vi "Bridge - Continuous Input.vi"() -> ()   [LabVIEW 2021]
doc: "This example demonstrates how to continuously acquire buffered bridge measurements (force/pressure/torque) using a DAQmx device.\n\nFor instructions on how to connect your signals to the DAQ device, refer to your device documentation."
uses:
  <vilib>/Utility/error.llb/DialogType.ctl
  <vilib>/DAQmx/read.llb/DAQmx Read (Analog 1D Wfm NChan NSamp).vi
  <vilib>/DAQmx/create/channels.llb/DAQmx Create Channel (AI-Force-Bridge-Two-Point-Linear).vi
  <vilib>/DAQmx/create/channels.llb/DAQmx Create Channel (AI-Force-Bridge-Table).vi
  <vilib>/DAQmx/create/channels.llb/DAQmx Create Channel (AI-Force-Bridge-Polynomial).vi
  <vilib>/DAQmx/create/channels.llb/DAQmx Create Channel (AI-Pressure-Bridge-Two-Point-Linear).vi
  <vilib>/DAQmx/create/channels.llb/DAQmx Create Channel (AI-Pressure-Bridge-Table).vi
  <vilib>/DAQmx/create/channels.llb/DAQmx Create Channel (AI-Pressure-Bridge-Polynomial).vi
  <vilib>/DAQmx/create/channels.llb/DAQmx Create Channel (AI-Torque-Bridge-Two-Point-Linear).vi
  <vilib>/DAQmx/create/channels.llb/DAQmx Create Channel (AI-Torque-Bridge-Table).vi
  <vilib>/DAQmx/create/channels.llb/DAQmx Create Channel (AI-Torque-Bridge-Polynomial).vi
  <vilib>/DAQmx/configure/timing.llb/DAQmx Timing (Sample Clock).vi
  <vilib>/DAQmx/configure/task.llb/DAQmx Configure Logging (TDMS).vi
  <vilib>/DAQmx/configure/trigger.llb/DAQmx Start Trigger (Digital Edge).vi
  <vilib>/DAQmx/configure/trigger.llb/DAQmx Start Trigger (Time).vi
  <vilib>/DAQmx/configure/trigger.llb/DAQmx Start Trigger (Analog Edge).vi
  <vilib>/DAQmx/calibration/calibrationInfo.llb/DAQmx Perform Shunt Calibration Ex (Bridge).vi
  <vilib>/DAQmx/miscellaneous.llb/DAQmx Fill In Error Info.vi
  <resource>/objmgr/daqmx.rc
panel:
  in  "Trigger Type":T1(tab)
  in  "Digital Start Trigger Edge":i32(ring)=10280 caption="Edge" items=["Rising"=10280, "Falling"=10171]
  in  "Digital Start Trigger Source":tag="/Dev1/PFI0" caption="Source"
  in  "Digital Pause Trigger Pause When":i32(ring)=10192 caption="Pause When" items=["High"=10192, "Low"=10214]
  in  "Digital Pause Trigger Source":tag="/Dev1/PFI0" caption="Source"
  in  "Analog Start Trigger Level":dbl caption="Level" format="%0.2f"
  in  "Analog Start Trigger Hysteresis":dbl caption="Hysteresis" format="%.2f"
  in  "Analog Start Trigger Slope":i32(ring)=10280 caption="Slope" items=["Rising"=10280, "Falling"=10171]
  in  "Analog Start Trigger Source":string="APFI0" caption="Source"
  in  "Analog Pause Trigger Source":string="APFI0" caption="Source"
  in  "Analog Pause Trigger Pause When":i32(ring)=10093 caption="Pause When" items=["Above Level"=10093, "Below Level"=10107]
  in  "Analog Pause Trigger Level":dbl caption="Level" format="%.2f"
  in  "When":timestamp
  in  "Select Time\nManually":bool
  in  "Logging Mode":i32(ring)=10231 items=["Off"=10231, "Log and Read"=15842]
  in  "TDMS File Path":path
  in  "Bridge Information":T2={"Bridge Configuration"=10182, "Excitation Source"=10200, "Excitation Value"=2.5, "Nominal Resistance"=350.0} {"Excitation Source" items=["Internal"=10200, "External"=10167, "None"=10230]; "Bridge Configuration" items=["Full Bridge"=10182, "Half Bridge"=10187, "Quarter Bridge"=10270, "No Bridge"=10228]}
  in  "Do Shunt Cal?":bool caption="Enable Shunt Cal"
  in  "Shunt Element Location":i32(ring)=12465 caption="shunt element location" items=["R1"=12465, "R2"=12466, "R3"=12467, "R4"=14813, "None"=10230]
  in  "Shunt Resistance":dbl=100000.0 format="%#.3p"
  in  "Do Offset Null?":bool caption="Enable Offset Null"
  in  "Physical Channel":tag="PXI2Slot4/ai0"
  in  "Channel Parameters":enum32{"Force", "Pressure", "Torque"}(tab)
  in  "Force Scaling Parameters":T3(tab)
  in  "Scaling Information":T4={"First Electrical Value"=0.0, "Second Electrical Value"=2.0, "Electrical Units"=15897, "First Physical Value"=0.0, "Second Physical Value"=100.0, "Physical Units"=15876} {"Electrical Units" items=["V/V"=15896, "mV/V"=15897]; "Physical Units" items=["Newtons"=15875, "Pounds"=15876, "kgf"=15877]}
  in  "Physical Units":i32(ring)=15876 items=["Newtons"=15875, "Pounds"=15876, "kgf"=15877]
  in  "Electrical Units":i32(ring)=15897 items=["V/V"=15896, "mV/V"=15897]
  in  "Electrical Values":dbl[](array[numeric])=[-2.0, 0.0, 2.0]
  in  "Physical Values":dbl[](array[numeric])=[-100.0, 0.0, 100.0]
  in  "Forward Coefficients":dbl[](array[numeric])=[0.0, 50.0] caption="Forward Coefficients (y = a0 + a1 * x + a2 * x^2 + ...)"
  in  "Electrical Min":dbl=-2.0
  in  "Electrical Max":dbl=2.0
  out "Generated Reverse Coefficients":dbl[](array[numeric]) caption="Generated Reverse Coefficients (x = b0 + b1 * y +b2 * y^2 + ...)"
  in  "Electrical Units":i32(ring)=15897 items=["V/V"=15896, "mV/V"=15897]
  in  "Physical Units":i32(ring)=15876 items=["Newtons"=15875, "Pounds"=15876, "kgf"=15877]
  in  "Reverse Coefficients":dbl[](array[numeric])=[0.0, 50.0] caption="Reverse Coefficients (x = b0 + b1 * y + b2 * y^2 + ...)"
  in  "Physical Min":dbl=-2.0
  in  "Physical Max":dbl=2.0
  out "Generated Forward Coefficients":dbl[](array[numeric]) caption="Generated Forward Coefficients (y= a0 + a1 * x + a2 *x^2 + ...)"
  in  "Electrical Units":i32(ring)=15897 items=["V/V"=15896, "mV/V"=15897]
  in  "Physical Units":i32(ring)=15876 items=["Newtons"=15875, "Pounds"=15876, "kgf"=15877]
  in  "Units (Force)":i32(ring)=15876 items=["Newtons"=15875, "Pounds"=15876, "kgf"=15877, "From Custom Scale"=10065]
  in  "Minimum Force":dbl=-100.0
  in  "Maximum Force":dbl=100.0
  in  "Pressure Scaling Parameters":T3(tab)
  in  "Scaling Information":T4={"First Electrical Value"=0.0, "Second Electrical Value"=2.0, "Electrical Units"=15897, "First Physical Value"=0.0, "Second Physical Value"=100.0, "Physical Units"=15879} {"Electrical Units" items=["V/V"=15896, "mV/V"=15897]; "Physical Units" items=["Pascals"=10081, "psi"=15879, "bar"=15880]}
  in  "Physical Units":i32(ring)=15879 items=["Pascals"=10081, "psi"=15879, "bar"=15880]
  in  "Electrical Values":dbl[](array[numeric])=[-2.0, 0.0, 2.0]
  in  "Electrical Units":i32(ring)=15897 items=["V/V"=15896, "mV/V"=15897]
  in  "Physical Values":dbl[](array[numeric])=[-100.0, 0.0, 100.0]
  in  "Forward Coefficients":dbl[](array[numeric])=[0.0, 50.0] caption="Forward Coefficients (y = a0 + a1 * x + a2 * x^2 + ...)"
  in  "Electrical Min":dbl=-2.0
  in  "Electrical Max":dbl=2.0
  out "Generated Reverse Coefficients":dbl[](array[numeric]) caption="Generated Reverse Coefficients (x = b0 + b1 * y +b2 * y^2 + ...)"
  in  "Electrical Units":i32(ring)=15897 items=["V/V"=15896, "mV/V"=15897]
  in  "Physical Units":i32(ring)=15879 items=["Pascals"=10081, "psi"=15879, "bar"=15880]
  out "Generated Forward Coefficients":dbl[](array[numeric])=[-9.457141359022379e-15, 0.019999999999999976] caption="Generated Forward Coefficients (y= a0 + a1 * x + a2 *x^2 + ...)"
  in  "Reverse Coefficients":dbl[](array[numeric])=[0.0, 50.0] caption="Reverse Coefficients (x = b0 + b1 * y + b2 * y^2 + ...)"
  in  "Physical Min":dbl=-100.0
  in  "Physical Max":dbl=100.0
  in  "Electrical Units":i32(ring)=15897 items=["V/V"=15896, "mV/V"=15897]
  in  "Physical Units":i32(ring)=15879 items=["Pascals"=10081, "psi"=15879, "bar"=15880]
  in  "Units (Pressure)":i32(ring)=15879 items=["Pascals"=10081, "psi"=15879, "bar"=15880, "From Custom Scale"=10065]
  in  "Minimum Pressure":dbl=-100.0
  in  "Maximum Pressure":dbl=100.0
  in  "Units (Torque)":i32(ring)=15883 items=["Nm"=15881, "oz-in"=15882, "lb-in"=15883, "lb-ft"=15884, "From Custom Scale"=10065]
  in  "Torque Scaling Parameters":T3(tab)
  in  "Scaling Information":T4={"First Electrical Value"=0.0, "Second Electrical Value"=2.0, "Electrical Units"=15897, "First Physical Value"=0.0, "Second Physical Value"=100.0, "Physical Units"=15883} {"Electrical Units" items=["V/V"=15896, "mV/V"=15897]; "Physical Units" items=["Nm"=15881, "oz-in"=15882, "lb-in"=15883, "lb-ft"=15884]}
  in  "Electrical Values":dbl[](array[numeric])=[-2.0, 0.0, 2.0]
  in  "Electrical Units":i32(ring)=15897 items=["V/V"=15896, "mV/V"=15897]
  in  "Physical Values":dbl[](array[numeric])=[-100.0, 0.0, 100.0]
  in  "Physical Units":i32(ring)=15883 items=["Nm"=15881, "oz-in"=15882, "lb-in"=15883, "lb-ft"=15884]
  in  "Forward Coefficients":dbl[](array[numeric])=[0.0, 50.0] caption="Forward Coefficients (y = a0 + a1 * x + a2 * x^2 + ...)"
  in  "Electrical Min":dbl=-2.0
  in  "Electrical Max":dbl=2.0
  out "Generated Reverse Coefficients":dbl[](array[numeric]) caption="Generated Reverse Coefficients (x = b0 + b1 * y +b2 * y^2 + ...)"
  in  "Electrical Units":i32(ring)=15897 items=["V/V"=15896, "mV/V"=15897]
  in  "Physical Units":i32(ring)=15883 items=["Nm"=15881, "oz-in"=15882, "lb-in"=15883, "lb-ft"=15884]
  out "Generated Forward Coefficients":dbl[](array[numeric]) caption="Generated Forward Coefficients (y= a0 + a1 * x + a2 *x^2 + ...)"
  in  "Reverse Coefficients":dbl[](array[numeric])=[0.0, 50.0] caption="Reverse Coefficients (x = b0 + b1 * y + b2 * y^2 + ...)"
  in  "Physical Min":dbl=-100.0
  in  "Physical Max":dbl=100.0
  in  "Electrical Units":i32(ring)=15897 items=["V/V"=15896, "mV/V"=15897]
  in  "Physical Units":i32(ring)=15883 items=["Nm"=15881, "oz-in"=15882, "lb-in"=15883, "lb-ft"=15884]
  in  "Minimum Torque":dbl=-100.0
  in  "Maximum Torque":dbl=100.0
  in  "Stop":bool
  out "Waveform Chart":waveform(dbl)[](graph)
  in  "Samples per Loop":i32=100
  in  "Sample Rate":dbl=1000.0
  out "Actual Sample Rate":dbl format="%0.2f"
  # "Channel Settings"
  # "Acquired Data"
  # "Timing Settings"
  # "Logging Settings"
  # "Trigger Settings"
  # "Shunt Calibration and Offset Null Settings"
  # "To enable triggers, select a tab above, and configure the settings.\n\nNot all hardware supports all trigger types. Refer to your device documentation for more information."
  # "This trigger type is not supported in continuous sample timing. \n\nRefer to your device documentation for more information on which triggers are supported."
  # "This trigger type is not supported in continuous sample timing. \n\nRefer to your device documentation for more information on which triggers are supported."
  # "If time is not manually set, task will begin after 10 seconds"
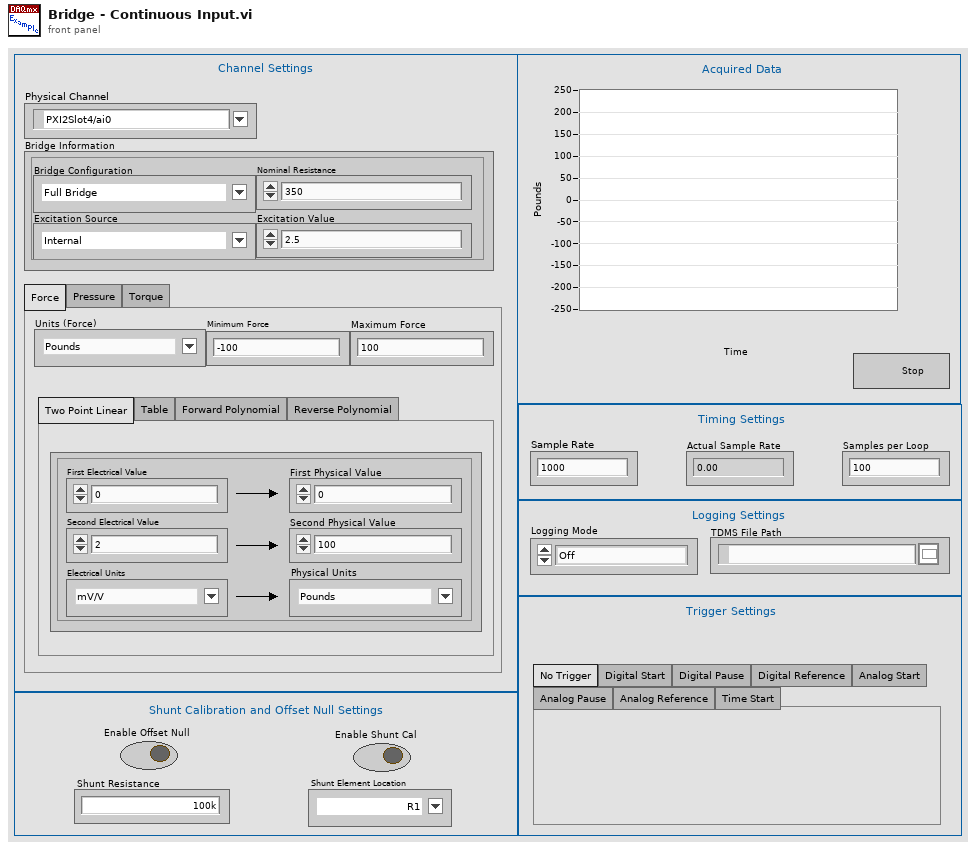
[diagram p1: front panel]
types:
  T1 = enum32{"No Trigger", "Digital Start", "Digital Pause", "Digital Reference", "Analog Start", "Analog Pause", "Analog Reference", "Time Start"}
  T2 = cluster{"Bridge Configuration":i32, "Excitation Source":i32, "Excitation Value":dbl, "Nominal Resistance":dbl}
  T3 = enum32{"Two Point Linear", "Table", "Forward Polynomial", "Reverse Polynomial"}
  T4 = cluster{"First Electrical Value":dbl, "Second Electrical Value":dbl, "Electrical Units":i32, "First Physical Value":dbl, "Second Physical Value":dbl, "Physical Units":i32}
  T5 = typedef "DialogType.ctl" = u16
  T6 = cluster{"Electrical Values":dbl[], "Electrical Units ":i32, "Physical Values":dbl[], "Physical Units  ":i32}
  T7 = cluster{"Forward Coefficients":dbl[], "reverse coefficients":dbl[], "Electrical Units":i32, "Physical Units":i32}
  T8 = cluster{"reverse coefficients":dbl[], "Reverse Coefficients":dbl[], "Electrical Units":i32, "Physical Units":i32}
  T9 = cluster{"Electrical Values":dbl[], "Electrical Units":i32, "Physical Values":dbl[], "Physical Units ":i32}
  T10 = cluster{"Electrical Values   ":dbl[], "Electrical Units    ":i32, "Physical Values  ":dbl[], "Physical Units":i32}
  T11 = cluster{"Forward Coefficients ":dbl[], "reverse coefficients":dbl[], "Electrical Units":i32, "Physical Units":i32}
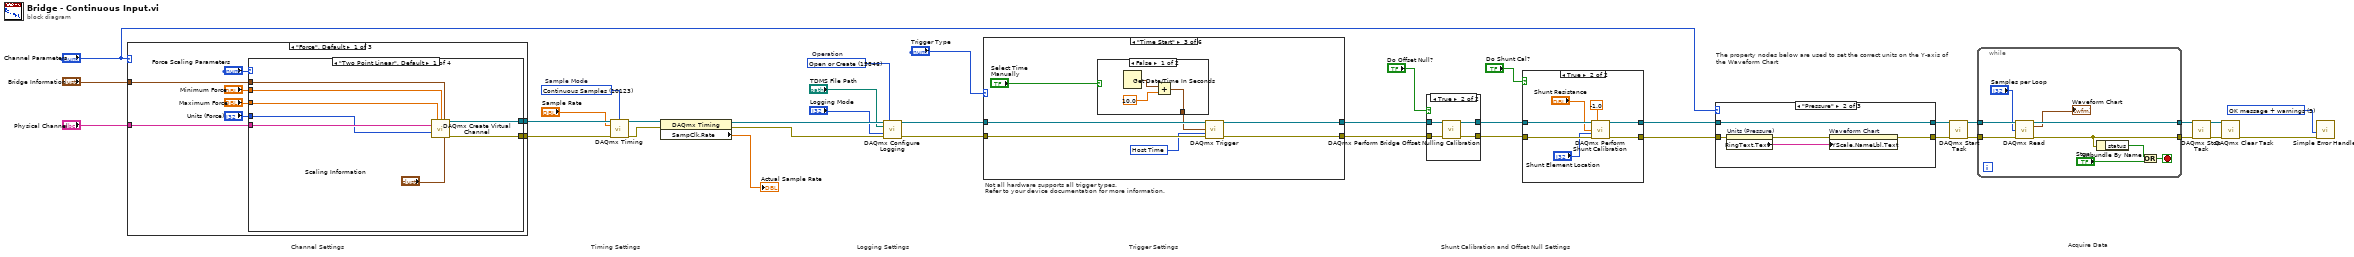
[diagram p0: block diagram]
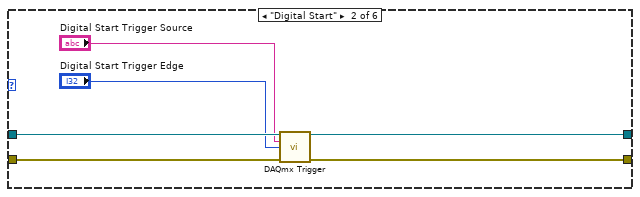
[diagram p3: hidden frame]
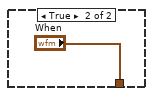
[diagram p4: hidden frame]
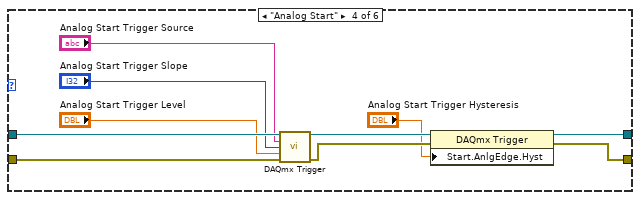
[diagram p5: hidden frame]
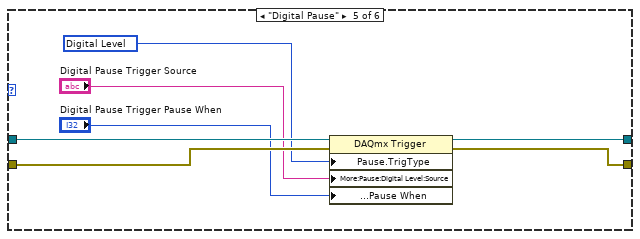
[diagram p6: hidden frame]
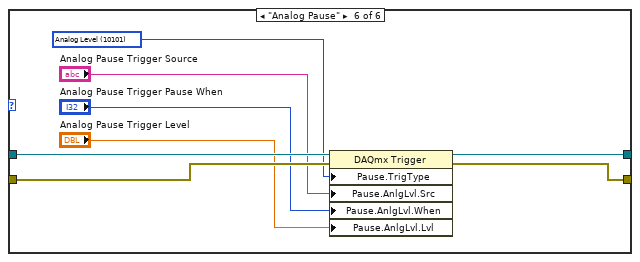
[diagram p7: hidden frame]
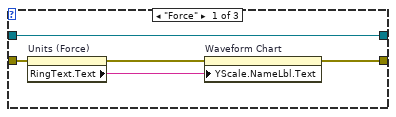
[diagram p8: hidden frame]
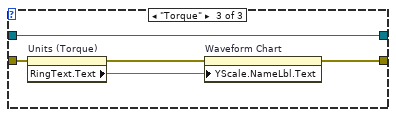
[diagram p9: hidden frame]
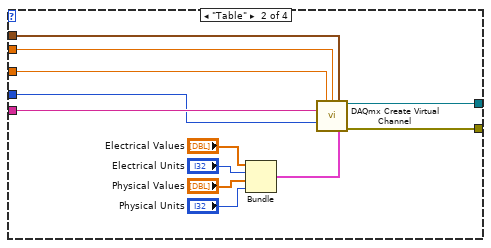
[diagram p12: hidden frame]
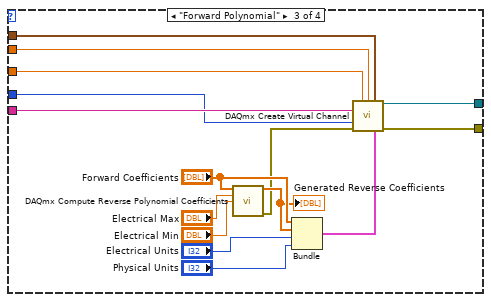
[diagram p13: hidden frame]
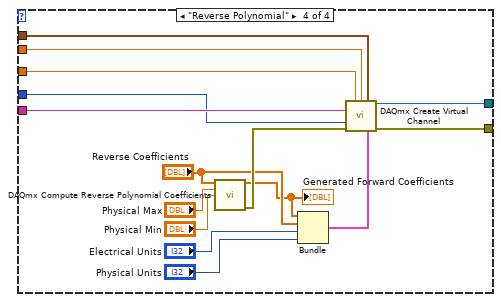
[diagram p14: hidden frame]
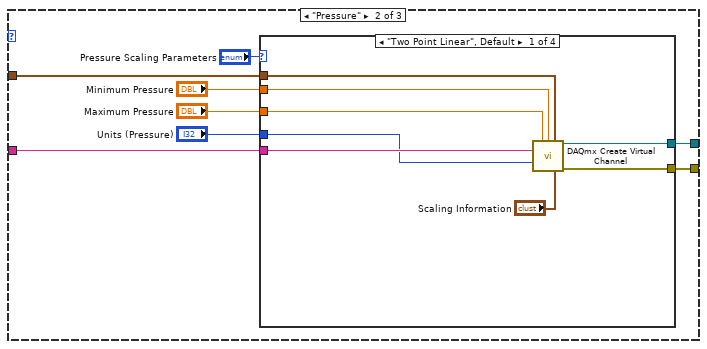
[diagram p15: hidden frame]
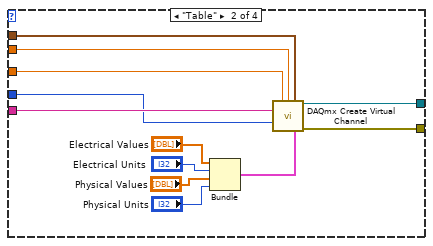
[diagram p16: hidden frame]
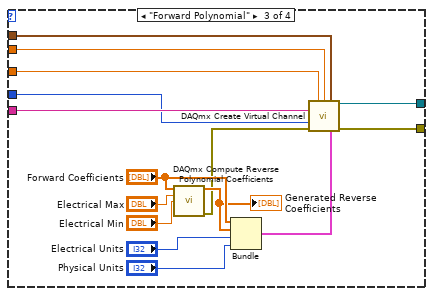
[diagram p17: hidden frame]
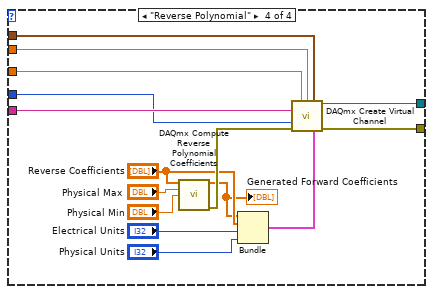
[diagram p18: hidden frame]
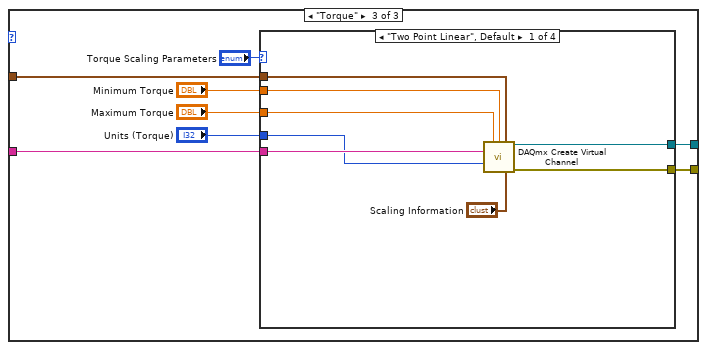
[diagram p19: hidden frame]
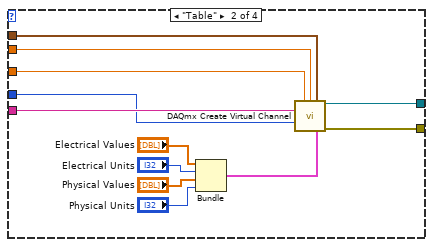
[diagram p20: hidden frame]
diagram:
  w6 = 15846 items=["Open"=10437, "Open or Create"=15846, "Create or Replace"=15847, "Create"=15848]  # Operation
  w10 = T5 3 items=["no dialog", "OK message", "continue or stop message", "OK message + warnings", "continue/stop + warnings"] ("type of dialog (OK msg:1)")
  w34 = 10123 items=["Finite Samples"=10178, "Continuous Samples"=10123, "Hardware Timed Single Point"=12522]  # Sample Mode
  # "Trigger Settings"
  # "Not all hardware supports all trigger types.\nRefer to your device documentation for more information."
  # "Logging Settings"
  # "The property nodes below are used to set the correct units on the Y-axis of the Waveform Chart"
  # "Acquire Data"
  # "Shunt Calibration and Offset Null Settings"
  # "Timing Settings"
  # "Channel Settings"
  n1 = case shown="\"Force\", Default" "Channel Parameters" {
    tunnel: [w41 w99 w157] -> w33
    tunnel: [w42 w100 w158] -> w32
    tunnel: "Physical Channel" -> [w43 w101 w159]
    tunnel: "Bridge Information" -> [w39 w97 w155]
    frame "Force", Default {
      n2 = case shown="\"Two Point Linear\", Default" "Force Scaling Parameters" {
        tunnel: w43 -> [w52 w64 w73 w93]
        tunnel: "Units (Force)" -> [w51 w63 w72 w92]
        tunnel: [w50 w62 w71 w91] -> w42
        tunnel: [w49 w61 w70 w90] -> w41
        tunnel: w39 -> [w47 w55 w67 w88]
        tunnel: "Minimum Force" -> [w46 w54 w66 w81]
        tunnel: "Maximum Force" -> [w45 w53 w65 w80]
        frame "Two Point Linear", Default {
          n3 = call-poly <vilib>:"DAQmx Create Virtual Channel.vi"("maximum value"=w45, "minimum value"=w46, "bridge information"=w47, "physical channels"=w52, "units"=w51, "scaling information"="Scaling Information") -> ("task out"=w50:refnum<k21>, "error out"=w49:errorcluster)  [unwired: 8 in]
        }
        frame "Table" {
          n4 = Bundle("Electrical Values"="Electrical Values", "Electrical Units"="Electrical Units", "Physical Values"="Physical Values", "Physical Units"="Physical Units") -> (w56:T6)  [unwired: 1 in]
          n5 = call-poly <vilib>:"DAQmx Create Virtual Channel.vi"("maximum value"=w53, "minimum value"=w54, "bridge information"=w55, "physical channels"=w64, "units"=w63, "scaling information"=w56) -> ("task out"=w62:refnum<k21>, "error out"=w61:errorcluster)  [unwired: 8 in]
        }
        frame "Forward Polynomial" {
          n6 = call <vilib>:"DAQmx Compute Reverse Polynomial Coefficients.vi"("coefficients"="Forward Coefficients", "maximum valid value of x"="Electrical Max", "minimum valid value of x"="Electrical Min") -> ("reverse coefficients"=w78:dbl[], "error out"=w75:errorcluster)  [unwired: 11 in]
          "Generated Reverse Coefficients" <- w78
          n7 = Bundle("Forward Coefficients"="Forward Coefficients", "reverse coefficients"=w78, "Electrical Units"="Electrical Units", "Physical Units"="Physical Units") -> (w74:T7)  [unwired: 1 in]
          n8 = call-poly <vilib>:"DAQmx Create Virtual Channel.vi"("maximum value"=w65, "minimum value"=w66, "bridge information"=w67, "physical channels"=w73, "units"=w72, "error in"=w75, "scaling information"=w74) -> ("task out"=w71:refnum<k21>, "error out"=w70:errorcluster)  [unwired: 7 in]
        }
        frame "Reverse Polynomial" {
          n9 = call <vilib>:"DAQmx Compute Reverse Polynomial Coefficients.vi"("coefficients"="Reverse Coefficients", "maximum valid value of x"="Physical Max", "minimum valid value of x"="Physical Min") -> ("reverse coefficients"=w86:dbl[], "error out"=w89:errorcluster)  [unwired: 11 in]
          "Generated Forward Coefficients" <- w86
          n10 = Bundle("reverse coefficients"=w86, "Reverse Coefficients"="Reverse Coefficients", "Electrical Units"="Electrical Units", "Physical Units"="Physical Units") -> (w94:T8)  [unwired: 1 in]
          n11 = call-poly <vilib>:"DAQmx Create Virtual Channel.vi"("maximum value"=w80, "minimum value"=w81, "bridge information"=w88, "physical channels"=w93, "units"=w92, "error in"=w89, "scaling information"=w94) -> ("task out"=w91:refnum<k21>, "error out"=w90:errorcluster)  [unwired: 7 in]
        }
      }
    }
    frame "Pressure" {
      n12 = case shown="\"Two Point Linear\", Default" "Pressure Scaling Parameters" {
        tunnel: w101 -> [w110 w122 w131 w149]
        tunnel: "Units (Pressure)" -> [w109 w121 w130 w148]
        tunnel: [w108 w120 w129 w147] -> w100
        tunnel: [w107 w119 w128 w146] -> w99
        tunnel: w97 -> [w105 w114 w125 w140]
        tunnel: "Minimum Pressure" -> [w104 w112 w124 w139]
        tunnel: "Maximum Pressure" -> [w103 w111 w123 w138]
        frame "Two Point Linear", Default {
          n13 = call-poly <vilib>:"DAQmx Create Virtual Channel.vi"("maximum value"=w103, "minimum value"=w104, "bridge information"=w105, "physical channels"=w110, "units"=w109, "scaling information"="Scaling Information") -> ("task out"=w108:refnum<k21>, "error out"=w107:errorcluster)  [unwired: 8 in]
        }
        frame "Table" {
          n14 = Bundle("Electrical Values"="Electrical Values", "Electrical Units"="Electrical Units", "Physical Values"="Physical Values", "Physical Units"="Physical Units") -> (w115:T9)  [unwired: 1 in]
          n15 = call-poly <vilib>:"DAQmx Create Virtual Channel.vi"("maximum value"=w111, "minimum value"=w112, "bridge information"=w114, "physical channels"=w122, "units"=w121, "scaling information"=w115) -> ("task out"=w120:refnum<k21>, "error out"=w119:errorcluster)  [unwired: 8 in]
        }
        frame "Forward Polynomial" {
          n16 = call <vilib>:"DAQmx Compute Reverse Polynomial Coefficients.vi"("coefficients"="Forward Coefficients", "maximum valid value of x"="Electrical Max", "minimum valid value of x"="Electrical Min") -> ("reverse coefficients"=w136:dbl[], "error out"=w133:errorcluster)  [unwired: 11 in]
          "Generated Reverse Coefficients" <- w136
          n17 = Bundle("Forward Coefficients"="Forward Coefficients", "reverse coefficients"=w136, "Electrical Units"="Electrical Units", "Physical Units"="Physical Units") -> (w132:T7)  [unwired: 1 in]
          n18 = call-poly <vilib>:"DAQmx Create Virtual Channel.vi"("maximum value"=w123, "minimum value"=w124, "bridge information"=w125, "physical channels"=w131, "units"=w130, "error in"=w133, "scaling information"=w132) -> ("task out"=w129:refnum<k21>, "error out"=w128:errorcluster)  [unwired: 7 in]
        }
        frame "Reverse Polynomial" {
          n19 = call <vilib>:"DAQmx Compute Reverse Polynomial Coefficients.vi"("coefficients"="Reverse Coefficients", "maximum valid value of x"="Physical Max", "minimum valid value of x"="Physical Min") -> ("reverse coefficients"=w141:dbl[], "error out"=w145:errorcluster)  [unwired: 11 in]
          "Generated Forward Coefficients" <- w141
          n20 = Bundle("reverse coefficients"=w141, "Reverse Coefficients"="Reverse Coefficients", "Electrical Units"="Electrical Units", "Physical Units"="Physical Units") -> (w150:T8)  [unwired: 1 in]
          n21 = call-poly <vilib>:"DAQmx Create Virtual Channel.vi"("maximum value"=w138, "minimum value"=w139, "bridge information"=w140, "physical channels"=w149, "units"=w148, "error in"=w145, "scaling information"=w150) -> ("task out"=w147:refnum<k21>, "error out"=w146:errorcluster)  [unwired: 7 in]
        }
      }
    }
    frame "Torque" {
      n22 = case shown="\"Two Point Linear\", Default" "Torque Scaling Parameters" {
        tunnel: w159 -> [w168 w180 w189 w207]
        tunnel: "Units (Torque)" -> [w167 w179 w188 w206]
        tunnel: [w166 w178 w187 w205] -> w158
        tunnel: [w165 w177 w186 w204] -> w157
        tunnel: w155 -> [w163 w171 w183 w198]
        tunnel: "Minimum Torque" -> [w162 w170 w182 w196]
        tunnel: "Maximum Torque" -> [w161 w169 w181 w197]
        frame "Two Point Linear", Default {
          n23 = call-poly <vilib>:"DAQmx Create Virtual Channel.vi"("maximum value"=w161, "minimum value"=w162, "bridge information"=w163, "physical channels"=w168, "units"=w167, "scaling information"="Scaling Information") -> ("task out"=w166:refnum<k21>, "error out"=w165:errorcluster)  [unwired: 8 in]
        }
        frame "Table" {
          n24 = Bundle("Electrical Values"="Electrical Values", "Electrical Units"="Electrical Units", "Physical Values"="Physical Values", "Physical Units"="Physical Units") -> (w172:T10)  [unwired: 1 in]
          n25 = call-poly <vilib>:"DAQmx Create Virtual Channel.vi"("maximum value"=w169, "minimum value"=w170, "bridge information"=w171, "physical channels"=w180, "units"=w179, "scaling information"=w172) -> ("task out"=w178:refnum<k21>, "error out"=w177:errorcluster)  [unwired: 8 in]
        }
        frame "Forward Polynomial" {
          n26 = call <vilib>:"DAQmx Compute Reverse Polynomial Coefficients.vi"("coefficients"="Forward Coefficients", "maximum valid value of x"="Electrical Max", "minimum valid value of x"="Electrical Min") -> ("reverse coefficients"=w194:dbl[], "error out"=w191:errorcluster)  [unwired: 11 in]
          "Generated Reverse Coefficients" <- w194
          n27 = Bundle("Forward Coefficients"="Forward Coefficients", "reverse coefficients"=w194, "Electrical Units"="Electrical Units", "Physical Units"="Physical Units") -> (w190:T11)  [unwired: 1 in]
          n28 = call-poly <vilib>:"DAQmx Create Virtual Channel.vi"("maximum value"=w181, "minimum value"=w182, "bridge information"=w183, "physical channels"=w189, "units"=w188, "error in"=w191, "scaling information"=w190) -> ("task out"=w187:refnum<k21>, "error out"=w186:errorcluster)  [unwired: 7 in]
        }
        frame "Reverse Polynomial" {
          n29 = call <vilib>:"DAQmx Compute Reverse Polynomial Coefficients.vi"("coefficients"="Reverse Coefficients", "maximum valid value of x"="Physical Max", "minimum valid value of x"="Physical Min") -> ("reverse coefficients"=w200:dbl[], "error out"=w203:errorcluster)  [unwired: 11 in]
          "Generated Forward Coefficients" <- w200
          n30 = Bundle("reverse coefficients"=w200, "Reverse Coefficients"="Reverse Coefficients", "Electrical Units"="Electrical Units", "Physical Units"="Physical Units") -> (w208:T8)  [unwired: 1 in]
          n31 = call-poly <vilib>:"DAQmx Create Virtual Channel.vi"("maximum value"=w197, "minimum value"=w196, "bridge information"=w198, "physical channels"=w207, "units"=w206, "error in"=w203, "scaling information"=w208) -> ("task out"=w205:refnum<k21>, "error out"=w204:errorcluster)  [unwired: 7 in]
        }
      }
    }
  }
  n32 = call-poly <vilib>:"DAQmx Timing.vi"("task/channels in"=w32, "sample mode"=w34, "rate"="Sample Rate", "error in"=w33) -> ("task out"=w36:refnum<k21>, "error out"=w35:errorcluster)  [unwired: 10 in]
  n33 = property class="DAQmx Timing"(reference=w36, error in=w35) -> (reference out=w9:refnum<k21>, error out=w16:errorcluster, "SampClk.Rate"=→"Actual Sample Rate":dbl)
  n34 = call-poly <vilib>:"DAQmx Configure Logging.vi"("task/channels in"=w9, "operation"=w6, "file path"="TDMS File Path", "logging mode"="Logging Mode", "error in"=w16) -> ("task out"=w2:refnum<k21>, "error out"=w1:errorcluster)  [unwired: 9 in]
  n35 = case shown="\"Time Start\"" "Trigger Type" {
    tunnel: w2 -> [w212 w218 w225 w239 w246 w254]
    tunnel: w1 -> [w211 w217 w224 w238 w243 w251]
    tunnel: [w212 w216 w223 w236 w245 w253] -> w3
    tunnel: [w211 w215 w222 w235 w244 w252] -> w4
    frame "No Trigger", Default {
    }
    frame "Digital Start" {
      n36 = call-poly <vilib>:"DAQmx Trigger.vi"("task/channels in"=w218, "source"="Digital Start Trigger Source", "edge"="Digital Start Trigger Edge", "error in"=w217) -> ("task out"=w216:refnum<k21>, "error out"=w215:errorcluster)  [unwired: 10 in]
    }
    frame "Time Start" {
      w219 = 16126 items=["Host Time"=16126, "I/O Device Time"=16127] ("timescale")
      n37 = case shown="False" "Select Time\nManually" {
        tunnel: [w228 "When"] -> w220
        frame False {
          n38 = Get Date/Time In Seconds() -> (seconds since 1Jan1904=w227:timestamp)
          n39 = Add(x=w227, y=10.0) -> (x+y=w228:timestamp)
        }
        frame True {
        }
      }
      n40 = call-poly <vilib>:"DAQmx Trigger.vi"("task/channels in"=w225, "when"=w220, "timescale"=w219, "error in"=w224) -> ("task out"=w223:refnum<k21>, "error out"=w222:errorcluster)  [unwired: 10 in]
    }
    frame "Analog Start" {
      n41 = call-poly <vilib>:"DAQmx Trigger.vi"("task/channels in"=w239, "source"="Analog Start Trigger Source", "slope"="Analog Start Trigger Slope", "level"="Analog Start Trigger Level", "error in"=w238) -> ("task out"=w234:refnum<k21>, "error out"=w233:errorcluster)  [unwired: 9 in]
      n42 = property class="DAQmx Trigger"(reference=w234, error in=w233, "Start.AnlgEdge.Hyst"="Analog Start Trigger Hysteresis") -> (reference out=w236:refnum<k21>, error out=w235:errorcluster)
    }
    frame "Digital Pause" {
      w242 = 10152 items=["Analog Level"=10101, "Analog Window"=10103, "Digital Level"=10152, "Digital Pattern"=10398, "None"=10230] ("Pause.TrigType")
      n43 = property class="DAQmx Trigger"(reference=w246, error in=w243, "Pause.TrigType"=w242, "More:Pause:Digital Level:Source"="Digital Pause Trigger Source", "More:Pause:Digital Level:Pause When"="Digital Pause Trigger Pause When") -> (reference out=w245:refnum<k21>, error out=w244:errorcluster)
    }
    frame "Analog Pause" {
      w250 = 10101 items=["Analog Level"=10101, "Analog Window"=10103, "Digital Level"=10152, "Digital Pattern"=10398, "None"=10230] ("Pause.TrigType")
      n44 = property class="DAQmx Trigger"(reference=w254, error in=w251, "Pause.TrigType"=w250, "Pause.AnlgLvl.Src"="Analog Pause Trigger Source", "Pause.AnlgLvl.When"="Analog Pause Trigger Pause When", "Pause.AnlgLvl.Lvl"="Analog Pause Trigger Level") -> (reference out=w253:refnum<k21>, error out=w252:errorcluster)
    }
  }
  n45 = case shown="True" "Do Offset Null?" {
    tunnel: [w256 w260] -> w24
    tunnel: [w255 w259] -> w23
    tunnel: w3 -> [w256 w258]
    tunnel: w4 -> [w255 w257]
    frame False {
    }
    frame True {
      n46 = call <vilib>:"DAQmx Perform Bridge Offset Nulling Calibration.vi"("task/channels in"=w258, "error in"=w257) -> ("task out"=w260:refnum<k21>, "error out"=w259:errorcluster)  [unwired: 12 in]
    }
  }
  n47 = case shown="True" "Do Shunt Cal?" {
    tunnel: w24 -> [w262 w269]
    tunnel: w23 -> [w261 w268]
    tunnel: [w261 w267] -> w22
    tunnel: [w262 w266] -> w18
    frame False {
    }
    frame True {
      n48 = call-poly <vilib>:"DAQmx Perform Shunt Calibration.vi"("task/channels in"=w269, "bridge resistance"=-1.0, "shunt resistance"="Shunt Resistance", "shunt element location"="Shunt Element Location", "error in"=w268) -> ("task out"=w266:refnum<k21>, "error out"=w267:errorcluster)  [unwired: 9 in]
    }
  }
  n49 = case shown="\"Pressure\"" "Channel Parameters" {
    tunnel: w22 -> [w274 w279 w284]
    tunnel: [w272 w277 w282] -> w21
    tunnel: [w270 w276 w283] -> w19
    tunnel: w18 -> [w270 w276 w283]
    frame "Force" {
      n50 = property on="Units (Force)" class="Ring (strict)"(error in=w274) -> (error out=w273:errorcluster, "RingText.Text"=w271:string)  [unwired: 1 in, 1 out]
      n51 = property on="Waveform Chart" class="WFChart (strict)"(error in=w273, "YScale.NameLbl.Text"=w271) -> (error out=w272:errorcluster)  [unwired: 1 in, 1 out]
    }
    frame "Pressure" {
      n52 = property on="Units (Pressure)" class="Ring (strict)"(error in=w279) -> (error out=w278:errorcluster, "RingText.Text"=w275:string)  [unwired: 1 in, 1 out]
      n53 = property on="Waveform Chart" class="WFChart (strict)"(error in=w278, "YScale.NameLbl.Text"=w275) -> (error out=w277:errorcluster)  [unwired: 1 in, 1 out]
    }
    frame "Torque" {
      n54 = property on="Units (Torque)" class="Ring (strict)"(error in=w284) -> (error out=w281:errorcluster, "RingText.Text"=w280:string)  [unwired: 1 in, 1 out]
      n55 = property on="Waveform Chart" class="WFChart (strict)"(error in=w281, "YScale.NameLbl.Text"=w280) -> (error out=w282:errorcluster)  [unwired: 1 in, 1 out]
    }
  }
  n56 = call <vilib>:"DAQmx Start Task.vi"("task/channels in"=w19, "error in"=w21) -> ("task out"=w31:refnum<k21>, "error out"=w30:errorcluster)  [unwired: 12 in]
  n57 = while {
    tunnel: w31 -> [w293]
    tunnel: w30 -> [w292]
    tunnel: [w289] -> w13
    tunnel: [w290] -> w14
    stop <- w291 stop-if-true
    n58 = call-poly <vilib>:"DAQmx Read.vi"("task/channels in"=w293, "number of samples per channel"="Samples per Loop", "error in"=w292) -> ("task out"=w290:refnum<k21>, "data"=→"Waveform Chart":waveform(dbl)[], "error out"=w289:errorcluster)  [unwired: 10 in]
    n59 = Unbundle By Name(w289) -> ("status"=w288:bool)
    n60 = Or(x=w288, y="Stop") -> (x .or. y?=w291:bool)
  }
  n61 = call <vilib>:"DAQmx Stop Task.vi"("task/channels in"=w14, "error in"=w13) -> ("task out"=w12:refnum<k21>, "error out"=w11:errorcluster)  [unwired: 12 in]
  n62 = call <vilib>:"DAQmx Clear Task.vi"("task in"=w12, "error in"=w11) -> ("error out"=w29:errorcluster)  [unwired: 13 in]
  n63 = call <vilib>:"Simple Error Handler.vi"("type of dialog (OK msg:1)"=w10, "error in (no error)"=w29) -> ()  [unwired: 3 in, 5 out]
